vi "Dynamic Dispatching.vi"   [LabVIEW 2010]
doc: "This example demonstrates dynamic dispatching with LabVIEW classes.\n\nRefer to the LabVIEW Help for more information about LabVIEW object-oriented programming."
uses:
  Vehicle/Vehicle.lvclass
panel:
  # "See block diagram for instructions."
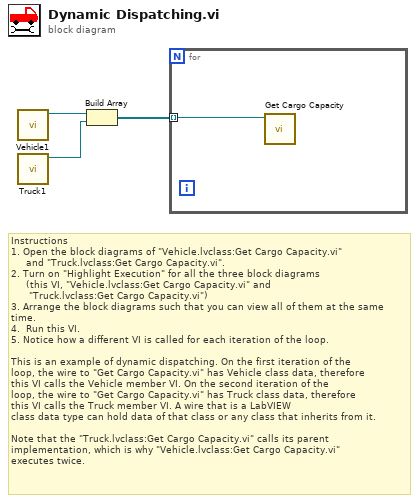
[diagram p0: block diagram]
diagram:
  # "Instructions\n1. Open the block diagrams of \"Vehicle.lvclass:Get Cargo Capacity.vi\"\n     and \"Truck.lvclass:Get Cargo Capacity.vi\".\n2. Turn on \"Highlight Execution\" for all the three block diagrams\n     (this VI, \"Vehicle.lvclass:Get Cargo Capacity.vi\" and \n      \"Truck.lvclass:Get Cargo Capacity.vi\")\n3. Arrange the block diagrams such that you can view all of them at the same time.\n4.  Run this VI.\n5. Notice how a different VI is called for each iteration of the loop.\n\nThis is an example of dynamic dispatching. On the first iteration of the\nloop, the wire to \"Get Cargo Capacity.vi\" has Vehicle class data, therefore\nthis VI calls the Vehicle member VI. On the second iteration of the\nloop, the wire to \"Get Cargo Capacity.vi\" has Truck class data, therefore\nthis VI calls the Truck member VI. A wire that is a LabVIEW \nclass data type can hold data of that class or any class that inherits from it.\n\nNote that the \"Truck.lvclass:Get Cargo Capacity.vi\" calls its parent\nimplementation, which is why \"Vehicle.lvclass:Get Cargo Capacity.vi\"\nexecutes twice."
  n1 = call "Vehicle1.vi"() -> ("vehicle"=w1:refnum<class "Vehicle.lvclass">)  [unwired: 11 in]
  n2 = call "Truck1.vi"() -> ("truck"=w3:refnum<class "Truck.lvclass">)  [unwired: 11 in]
  n3 = Build Array "Build Array"(w1, w3) -> (w2:refnum<class "Vehicle.lvclass">[])
  n4 = for {
    tunnel: w2 -> [w4] mode=indexing
    n5 = call-dynamic "Get Cargo Capacity.vi"("vehicle"=w4) -> ()  [unwired: 9 in, 2 out]
  }
